vi "setVDCLinkToPower.vi"(0 "Interface in":T4, 5 "VDCLinkToPower":T1={"gains"={"proportional gain"=0.0, "integral gain"=0.0}, "output range"={"output high (Inf)"=inf, "output low (-Inf)"=-inf}, "PI_state"=enum."idle", "reset"=FALSE, "manual"=0.0} {"gains"."proportional gain" step=0.125}, 11 "error in":errorcluster) -> (4 "Interface out":T4, 15 "error out":errorcluster)   [LabVIEW 2017, in "AFE_interface.lvlib"]
uses:
  AFE_interface.lvlib
  InterfaceRef.ctl
  <instrlib>/_niInstr/Instruction Framework/v1/Host/Instruction Target/niInstr Instruction Target v1 Host.lvclass
  <instrlib>/_niInstr/Instruction Framework/v1/Host/Instruction Framework Context/niInstr Instruction Framework Context v1 Host.lvclass
  AFE/PI_Settings.ctl
  <vilib>/rvi/Analysis/control/PID/Typedef/niFpgaPID_PIGains.ctl
  <vilib>/rvi/Analysis/control/PID/Typedef/niFpgaPID_OutputRange.ctl
  AFE/ActiveFrontEnd.lvlib
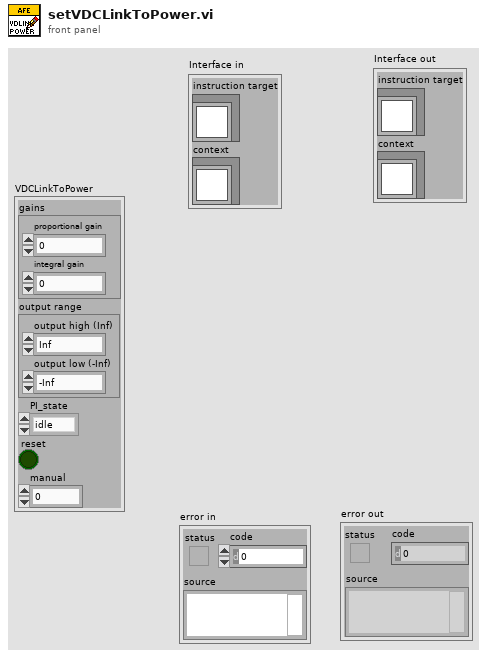
[diagram p1: front panel]
types:
  T1 = typedef "ActiveFrontEnd.lvlib/PI_Settings.ctl" = cluster{"gains":T2, "output range":T3, "PI_state":enum8{"idle", "normal", "manual", "perturbance"}, "reset":bool, "manual":sgl}
  T2 = typedef "niFpgaPID_PIGains.ctl" = cluster{"proportional gain":sgl, "integral gain":sgl}
  T3 = typedef "niFpgaPID_OutputRange.ctl" = cluster{"output high (Inf)":sgl, "output low (-Inf)":sgl}
  T4 = typedef "AFE_interface.lvlib/InterfaceRef.ctl" = cluster{"instruction target":refnum<class "niInstr Instruction Target v1 Host.lvclass">, "context":refnum<class "niInstr Instruction Framework Context v1 Host.lvclass">}
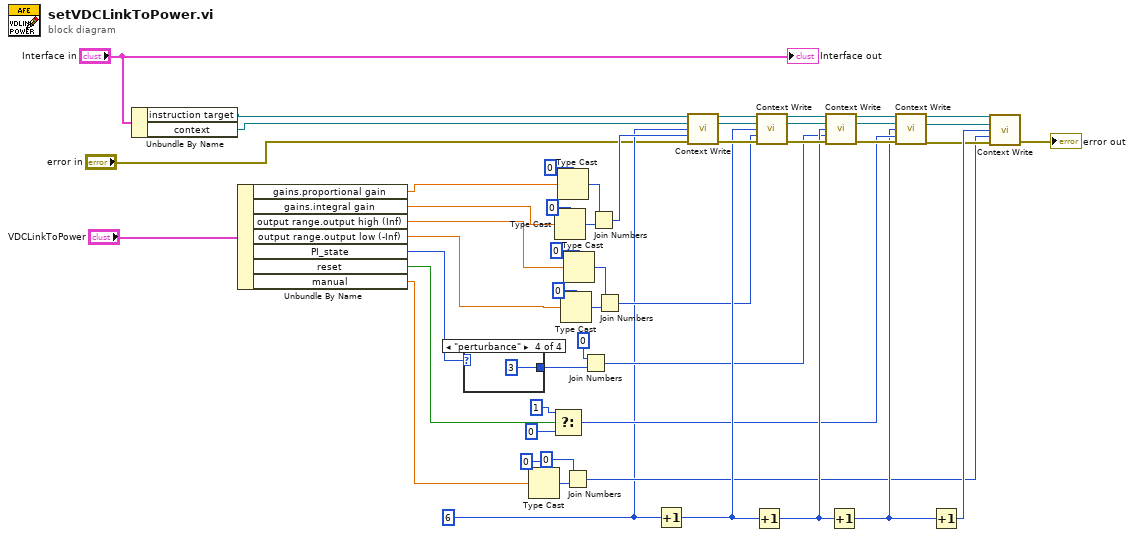
[diagram p0: block diagram]
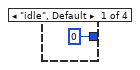
[diagram p2: hidden frame]
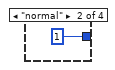
[diagram p3: hidden frame]
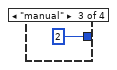
[diagram p4: hidden frame]
diagram:
  w3 = 6 ("x")
  n1 = Unbundle By Name("Interface in") -> ("instruction target"=w5:refnum<class "niInstr Instruction Target v1 Host.lvclass">, "context"=w4:refnum<class "niInstr Instruction Framework Context v1 Host.lvclass">)
  n2 = Unbundle By Name("VDCLinkToPower") -> ("gains.proportional gain"=w35:sgl, "gains.integral gain"=w34:sgl, "output range.output high (Inf)"=w28:sgl, "output range.output low (-Inf)"=w27:sgl, "PI_state"=w9:enum8{"idle", "normal", "manual", "perturbance"}, "reset"=w26:bool, "manual"=w12:sgl)
  n3 = case shown="\"perturbance\"" w9 {
    tunnel: [u32 0 u32 1 u32 2 u32 3] -> w8
    frame "idle", Default {
    }
    frame "normal" {
    }
    frame "manual" {
    }
    frame "perturbance" {
    }
  }
  n4 = Type Cast(type=u32 0, x=w12) -> (*(type *) &x=w14:u32)
  n5 = Select(t=u64 1 ("data"), s=w26, f=u64 0) -> (s? t:f=w21:u64)
  n6 = Type Cast(type=u32 0, x=w34) -> (*(type *) &x=w36:u32)
  n7 = Type Cast(type=u32 0, x=w35) -> (*(type *) &x=w39:u32)
  n8 = Type Cast(type=u32 0, x=w27) -> (*(type *) &x=w32:u32)
  n9 = Join Numbers(hi=u32 0, lo=w14) -> ((hi.lo)=w10:u64)
  n10 = Type Cast(type=u32 0, x=w28) -> (*(type *) &x=w29:u32)
  n11 = Join Numbers(hi=u32 0, lo=w8) -> ((hi.lo)=w24:u64)
  n12 = Join Numbers(hi=w39, lo=w36) -> ((hi.lo)=w33:u64)
  n13 = Join Numbers(hi=w29, lo=w32) -> ((hi.lo)=w25:u64)
  n14 = Increment(x=w3) -> (x+1=w41:i32)
  n15 = call <instrlib>:"Context Write.vi"("instruction target in"=w5, "context in"=w4, "address"=w3, "data"=w33, "error in"="error in") -> ("instruction target out"=w50:refnum<class "niInstr Instruction Target v1 Host.lvclass">, "context out"=w47:refnum<class "niInstr Instruction Framework Context v1 Host.lvclass">, "error out"=w44:errorcluster)  [unwired: 8 in]
  n16 = Increment(x=w41) -> (x+1=w40:i32)
  n17 = call <instrlib>:"Context Write.vi"("instruction target in"=w50, "context in"=w47, "address"=w41, "data"=w25, "error in"=w44) -> ("instruction target out"=w49:refnum<class "niInstr Instruction Target v1 Host.lvclass">, "context out"=w46:refnum<class "niInstr Instruction Framework Context v1 Host.lvclass">, "error out"=w43:errorcluster)  [unwired: 8 in]
  n18 = call <instrlib>:"Context Write.vi"("instruction target in"=w49, "context in"=w46, "address"=w40, "data"=w24, "error in"=w43) -> ("instruction target out"=w48:refnum<class "niInstr Instruction Target v1 Host.lvclass">, "context out"=w45:refnum<class "niInstr Instruction Framework Context v1 Host.lvclass">, "error out"=w42:errorcluster)  [unwired: 8 in]
  n19 = Increment(x=w40) -> (x+1=w19:i32)
  n20 = call <instrlib>:"Context Write.vi"("instruction target in"=w48, "context in"=w45, "address"=w19, "data"=w21, "error in"=w42) -> ("instruction target out"=w17:refnum<class "niInstr Instruction Target v1 Host.lvclass">, "context out"=w16:refnum<class "niInstr Instruction Framework Context v1 Host.lvclass">, "error out"=w15:errorcluster)  [unwired: 8 in]
  n21 = Increment(x=w19) -> (x+1=w18:i32)
  n22 = call <instrlib>:"Context Write.vi"("instruction target in"=w17, "context in"=w16, "address"=w18, "data"=w10, "error in"=w15) -> ("error out"=→"error out":errorcluster)  [unwired: 8 in, 2 out]
  "Interface out" <- "Interface in"
